vi "array FOLI.vi"(9 "status string":string, 11 "Megger cluster in":T1={"Read data"={"Firmware version"="", "Model number"="", "Serial number"=0, "Ramp rate"=0.0, "Test Voltage"=0.0, "Test duration"=0.0, "Test stop watch"=0.0, "measured Current (nA)"=0.0, "calculated Resistance"=0.0, "Test Mode"=enum."Insulation resistance (IR)", "Test status"=enum."Waiting to start test"}, "Connected?"=FALSE, "Device status array"=[]}) -> (3 "Megger cluster out":T1={"Read data"={"Firmware version"="", "Model number"="", "Serial number"=0, "Ramp rate"=0.0, "Test Voltage"=0.0, "Test duration"=0.0, "Test stop watch"=0.0, "measured Current (nA)"=0.0, "calculated Resistance"=0.0, "Test Mode"=enum."Insulation resistance (IR)", "Test status"=enum."Waiting to start test"}, "Connected?"=FALSE, "Device status array"=[]})   [LabVIEW 2014]
uses:
  Controls/Megger cluster.ctl
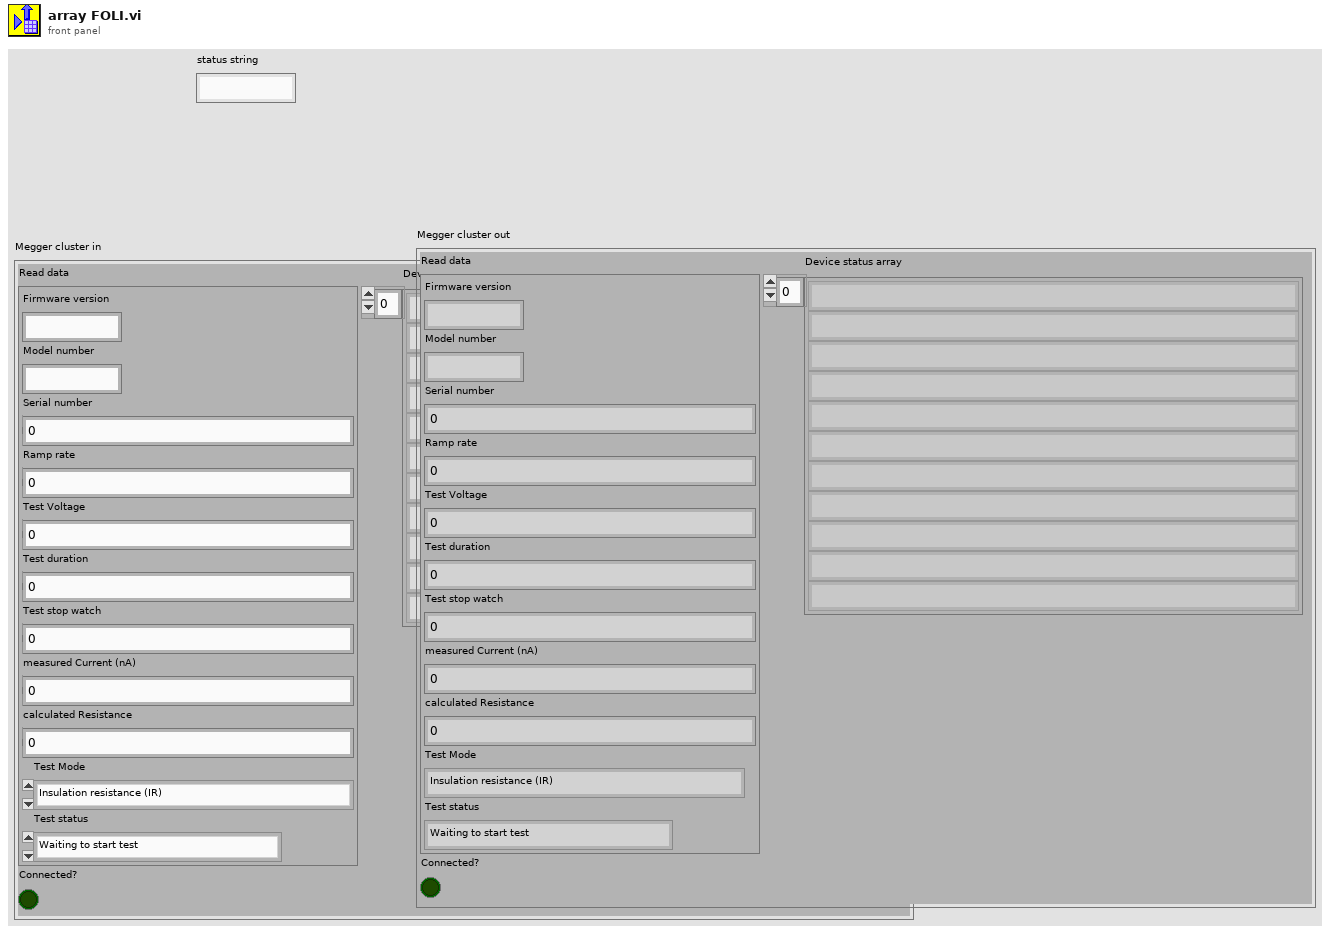
[diagram p1: front panel]
types:
  T1 = typedef "Megger cluster.ctl" = cluster{"Read data":cluster{"Firmware version":string, "Model number":string, "Serial number":i32, "Ramp rate":dbl, "Test Voltage":dbl, "Test duration":sgl, "Test stop watch":sgl, "measured Current (nA)":dbl, "calculated Resistance":dbl, "Test Mode":enum16{"N/A", "Insulation resistance (IR)", "Timed Insulation resistance (IR(t))", "Diaelectric Absorption Ratio (DAR)", "Polarisation Index (PI)", "Diaelectric Dishcharge (DD)", "Step voltage (SV)", "Ramp test (Ramp)"}, "Test status":enum16{"Waiting to start test", "Unable to start test", "Test progressing normally", "Performing post test measurements", "Test has ended normally", "Test has been aborted"}}, "Connected?":bool, "Device status array":string[]}
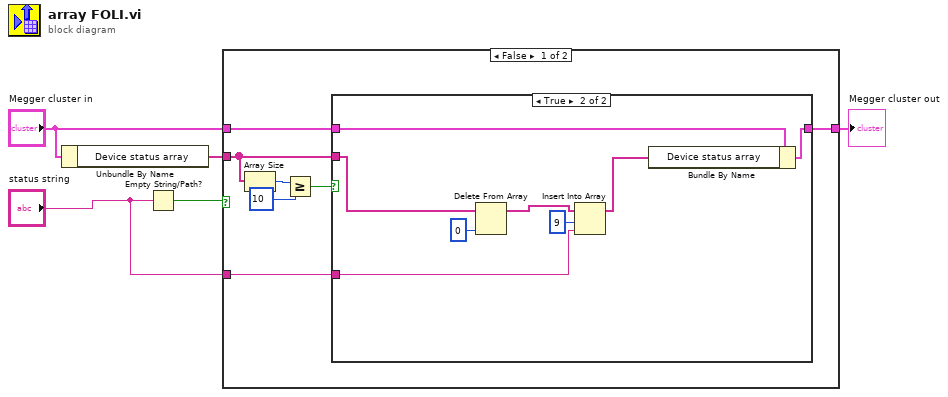
[diagram p0: block diagram]
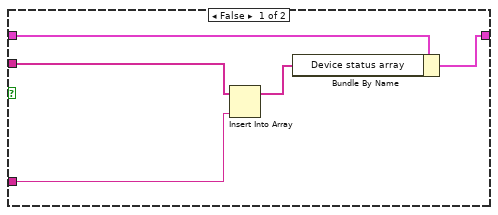
[diagram p2: hidden frame]
diagram:
  n1 = Unbundle By Name("Megger cluster in") -> ("Device status array"=w3:string[])
  n2 = Empty String/Path?(string/path="status string") -> (empty?=w5:bool)
  n3 = case shown="False" w5 {
    tunnel: "Megger cluster in" -> [w12 w26]
    tunnel: [w11 w26] -> w1
    tunnel: w3 -> [w10 _]
    tunnel: "status string" -> [w7 _]
    frame False {
      n4 = Array Size(array=w10) -> (size(s)=w9:i32)
      n5 = Greater Or Equal?(x=w9, y=10) -> (x >= y?=w8:bool)
      n6 = case shown="True" w8 {
        tunnel: w12 -> [w15 w25]
        tunnel: [w14 w24] -> w11
        tunnel: w10 -> [w16 w19]
        tunnel: w7 -> [w17 w20]
        frame False {
          n7 = Insert Into Array(array=w16, new element=w17) -> (w13:string[])  [unwired: 1 in]
          n8 = Bundle By Name(cluster=w15, "Device status array"=w13) -> (w14:T1)
        }
        frame True {
          n9 = Delete From Array(array=w19, index=0) -> (array with subset deleted=w21:string[])  [unwired: 1 in, 1 out]
          n10 = Insert Into Array(array=w21, index=9, new element=w20) -> (w18:string[])
          n11 = Bundle By Name(cluster=w25, "Device status array"=w18) -> (w24:T1)
        }
      }
    }
    frame True {
    }
  }
  "Megger cluster out" <- w1
